vi "Create.vi"(8 "error in (no error)":errorcluster, 10 "mqtt instance":refnum<class "MQTT Client.lvclass">) -> (0 "error out":errorcluster, 3 "mqttCmdConnect out":refnum<class "ConnectMqttMsg.lvclass">)   [LabVIEW 2020, in "ConnectMqttMsg.lvclass"]
uses:
  ConnectMqttMsg.lvclass
  MQTT Client.lvclass
  ConnectMqttMsg.lvclass/ConnectMqttMsg.ctl
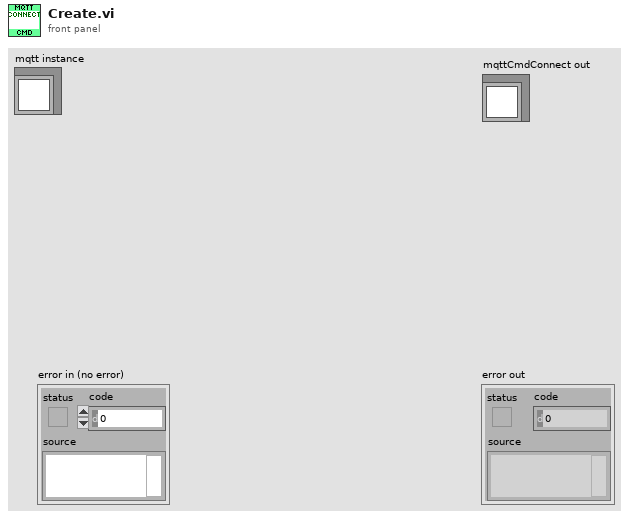
[diagram p1: front panel]
types:
  T1 = typedef "MQTT Client.lvclass/ConnectionConfig.ctl" = cluster{"Client ID":string, "Host":string, "Port":u16, "Connection Timeout":i32, "Write Timeout":i32, "Read Timeout":i32, "Sub Timeout":i32, "Keep Alive (sec)":u16, "Clean Session":bool, "Use TLS":bool}
  T2 = typedef "MQTT Client.lvclass/ConnectionFlags.ctl" = cluster{"user name":bool, "password":bool, "will retain":bool, "will flag":bool, "clean session":bool, "reserved":bool, "willQOS":T3}
  T3 = typedef "BaseMqttMsg.lvclass/QosLevel.ctl" = enum8{"At most once", "At least once", "Exactly once", "Reserved"}
  T4 = typedef "MQTT Client.lvclass/UserCredentials.ctl" = cluster{"User Name":string, "Password":string}
  T5 = typedef "MQTT Client.lvclass/WillDefinition.ctl" = cluster{"Will Topic":string, "Will message":string, "connMeta":T6}
  T6 = typedef "MQTT Client.lvclass/ConnectionMeta.ctl" = cluster{"qos":T3, "duplicate":bool, "retain":bool}
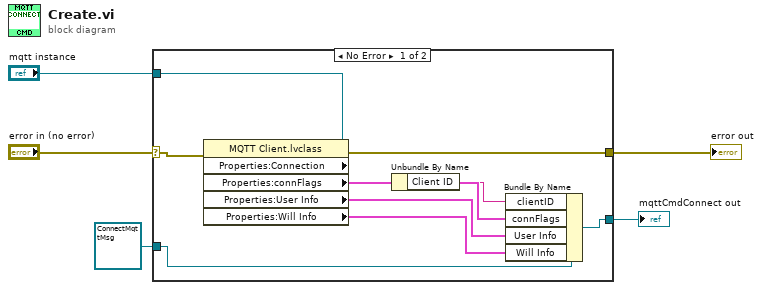
[diagram p0: block diagram]
diagram:
  n1 = case shown="No Error" "error in (no error)" {
    selector: "error in (no error)" -> [w13 w17]
    tunnel: [w14 w17] -> w4
    tunnel: [w7 w16] -> w1
    tunnel: "mqtt instance" -> [w15 _]
    tunnel: refnum<class "ConnectMqttMsg.lvclass"> refnum ("mqttCmdConnect out") -> [w12 w16]
    frame No Error {
      n2 = property class="MQTT Client.lvclass"(reference=w15, error in=w13) -> (error out=w14:errorcluster, "Properties:Connection"=w11:T1, "Properties:connFlags"=w10:T2, "Properties:User Info"=w9:T4, "Properties:Will Info"=w8:T5)  [unwired: 1 out]
      n3 = Unbundle By Name(w11) -> ("Client ID"=w6:string)
      n4 = Bundle By Name(cluster=w12, "clientID"=w6, "connFlags"=w10, "User Info"=w9, "Will Info"=w8) -> (w7:refnum<class "ConnectMqttMsg.lvclass">)
    }
    frame Error {
    }
  }
  "error out" <- w4
  "mqttCmdConnect out" <- w1
